vi "AOTFSetPosition.vi"   [LabVIEW 2009]
uses:
  AO Update Channel (scaled value).vi
types:
  T1 = typedef "AnalogSettings.ctt" = cluster{"PCI 671x Device Number":u32, "Samples per Unit":u32}
  T2 = typedef "AOTFSettings.ctt" = cluster{"Laser 1 Output Channel":tag, "AOTF  1 Output Voltage":dbl, "Laser 2 Output Channel":tag, "AOTF  2 Output Voltage":dbl, "Laser 3 Output Channel":tag, "AOTF  3 Output Voltage":dbl, "Pixel per Cycle":u16, "Time per Cycle  / ms":dbl, "Laser 4 Output Channel":tag, "AOTF  4 Output Voltage":dbl, "Laser 5 Output Channel":tag, "AOTF 5 Output Voltage ":dbl, "Laser 6 Output Channel":tag, "AOTF  6 Output Voltage ":dbl, "Laser 7 Output Channel":tag, "AOTF 7 Output Voltage ":dbl, "Laser 8 Output Channel":tag, "AOTF  8 Output Voltage ":dbl, "AOTF  1 Frequency":dbl, "AOTF  2 Frequency":dbl, "AOTF  3  Frequency":dbl, "AOTF  4 Frequency":dbl, "AOTF 5 Frequency":dbl, "AOTF  6 Frequency":dbl, "AOTF 7  Frequency":dbl, "AOTF  8 Frequency":dbl, "AOTF  1 Amplitude":dbl, "AOTF  2 Amplitude":dbl, "AOTF  3  Amplitude":dbl, "AOTF  4 Amplitude":dbl, "AOTF 5 Amplitude":dbl, "AOTF  6 Amplitude":dbl, "AOTF 7 Amplitude  ":dbl, "AOTF  8 Amplitude":dbl}
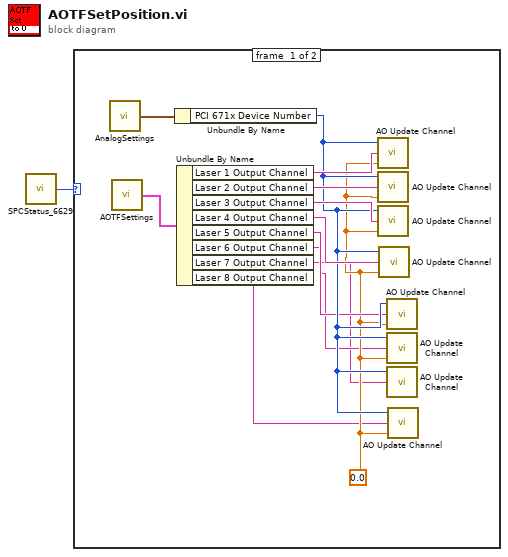
[diagram p0: block diagram]
diagram:
  n1 = call "SPCStatus_6629.vi"() -> ("Status (output)"=w1:enum16{"offline", "online", "busy"})  [unwired: 2 in]
  n2 = case shown="\"offline\", Default" w1 {
    frame #0 {
      w5 = sgl 0.0 ("value")
      n3 = call "AnalogSettings.vi"() -> ("Analog Settings (output)"=w9:T1)  [unwired: 2 in]
      n4 = call "AOTFSettings.vi"() -> ("AOTF Setting (Output)"=w13:T2)  [unwired: 2 in]
      n5 = Unbundle By Name(w9) -> ("PCI 671x Device Number"=w7:u32)
      n6 = Unbundle By Name(w13) -> ("Laser 1 Output Channel"=w11:tag, "Laser 2 Output Channel"=w12:tag, "Laser 3 Output Channel"=w10:tag, "Laser 4 Output Channel"=w8:tag, "Laser 5 Output Channel"=w6:tag, "Laser 6 Output Channel"=w4:tag, "Laser 7 Output Channel"=w3:tag, "Laser 8 Output Channel"=w2:tag)
      n7 = call-poly "AO Update Channel.vi"("value"=w5, "channel (0)"=w11, "device"=w7) -> ()
      n8 = call-poly "AO Update Channel.vi"("value"=w5, "channel (0)"=w12, "device"=w7) -> ()
      n9 = call-poly "AO Update Channel.vi"("value"=w5, "channel (0)"=w10, "device"=w7) -> ()
      n10 = call-poly "AO Update Channel.vi"("value"=w5, "channel (0)"=w8, "device"=w7) -> ()
      n11 = call-poly "AO Update Channel.vi"("value"=w5, "channel (0)"=w6, "device"=w7) -> ()
      n12 = call-poly "AO Update Channel.vi"("value"=w5, "channel (0)"=w4, "device"=w7) -> ()
      n13 = call-poly "AO Update Channel.vi"("channel (0)"=w3, "device"=w7) -> ()  [unwired: 1 in]
      n14 = call-poly "AO Update Channel.vi"("value"=w5, "channel (0)"=w2, "device"=w7) -> ()
    }
    frame #1 {
    }
  }
